vi "Read max pressure.vi"(8 "error in (no error)":errorcluster, 11 "Component-B in":refnum<class "Component-B.lvclass">) -> (0 "error out":errorcluster, 2 "max pressure":dbl, 3 "Component-B out":refnum<class "Component-B.lvclass">)   [LabVIEW 2018, in "Component-B.lvclass"]
uses:
  Component-B.lvclass
  Component-B.lvclass/Component-B.ctl
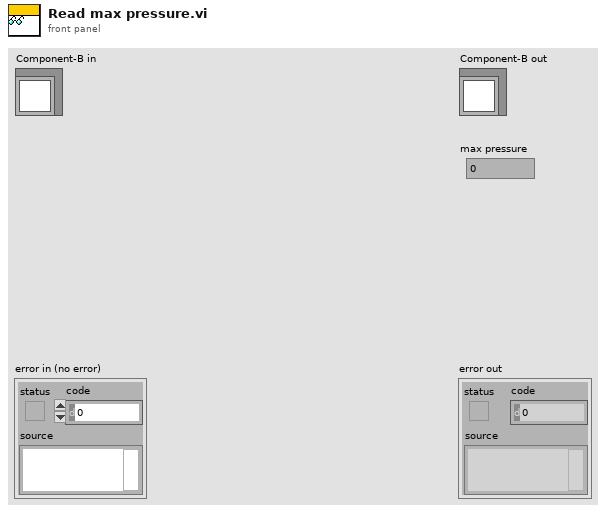
[diagram p1: front panel]
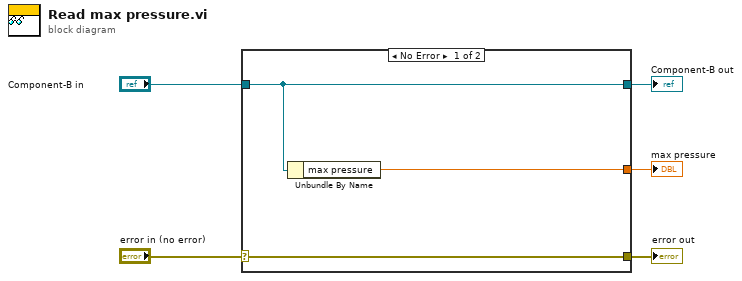
[diagram p0: block diagram]
diagram:
  n1 = case shown="No Error" "error in (no error)" {
    selector: "error in (no error)" -> [w8 w9]
    tunnel: [w8 w9] -> w4
    tunnel: [w7 w10] -> w2
    tunnel: "Component-B in" -> [w7 w10]
    tunnel: [w6 _] -> w1
    frame No Error {
      n2 = Unbundle By Name(w7) -> ("max pressure"=w6:dbl)
    }
    frame Error {
    }
  }
  "error out" <- w4
  "Component-B out" <- w2
  "max pressure" <- w1
